vi "Close SHVs.vi"(8 "error in (no error)":errorcluster, 11 "Heater in":refnum<class "Heater.lvclass">) -> (0 "error out":errorcluster, 3 "Heater out":refnum<class "Heater.lvclass">)   [LabVIEW 2015, in "cRIO-Carbondioxide.lvlib" / "CO2-Actor.lvlib" / "Heater.lvclass"]
uses:
  Heater.lvclass
  Heater.lvclass/Heater.ctl
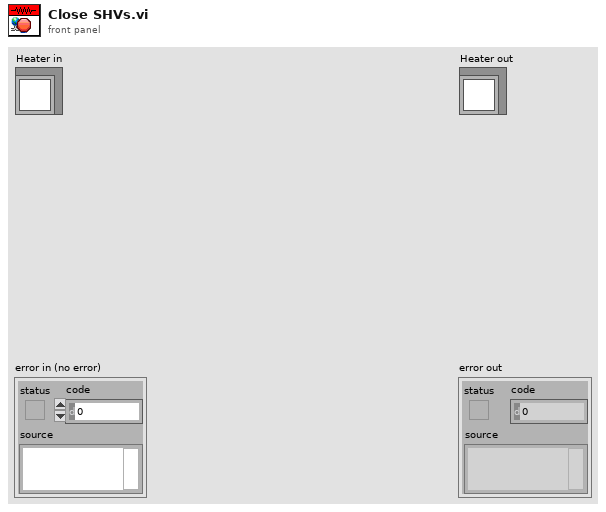
[diagram p1: front panel]
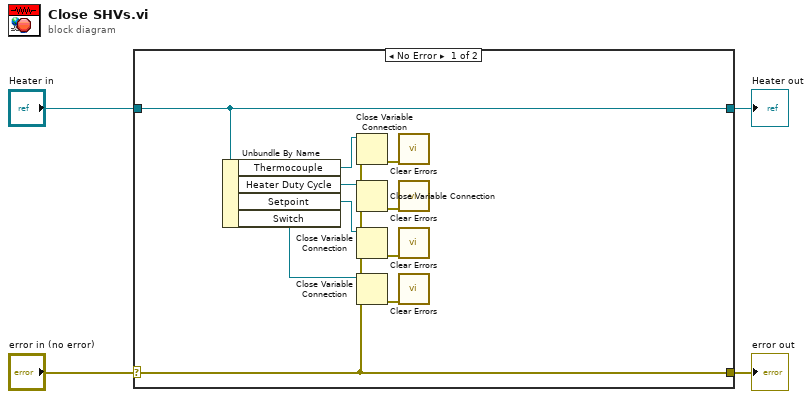
[diagram p0: block diagram]
diagram:
  n1 = case shown="No Error" "error in (no error)" {
    selector: "error in (no error)" -> [w6 w16]
    tunnel: [w6 w16] -> w3
    tunnel: [w8 w15] -> w1
    tunnel: "Heater in" -> [w8 w15]
    frame No Error {
      n2 = Unbundle By Name(w8) -> ("Thermocouple"=w11:refnum<k21>, "Heater Duty Cycle"=w13:refnum<k21>, "Setpoint"=w9:refnum<k21>, "Switch"=w5:refnum<k21>)
      n3 = Close Variable Connection(8:w6, 11:w11) -> (0:w10:errorcluster)
      n4 = Close Variable Connection(8:w6, 11:w13) -> (0:w12:errorcluster)
      n5 = Close Variable Connection(8:w6, 11:w9) -> (0:w14:errorcluster)
      n6 = Close Variable Connection(8:w6, 11:w5) -> (0:w7:errorcluster)
      n7 = call <vilib>:"Clear Errors.vi"("error in (no error)"=w10) -> ()  [unwired: 5 in, 2 out]
      n8 = call <vilib>:"Clear Errors.vi"("error in (no error)"=w12) -> ()  [unwired: 5 in, 2 out]
      n9 = call <vilib>:"Clear Errors.vi"("error in (no error)"=w14) -> ()  [unwired: 5 in, 2 out]
      n10 = call <vilib>:"Clear Errors.vi"("error in (no error)"=w7) -> ()  [unwired: 5 in, 2 out]
    }
    frame Error {
    }
  }
  "error out" <- w3
  "Heater out" <- w1
